vi "Save-OsciVsTime.vi"(0 "X-Values":dbl[](array[numeric]) format="%.2f", 2 "error in":errorcluster, 3 "Y-Values":dbl[](array[numeric]) format="%.2f", 4 "comment":string, 5 "refnum":refnum<file>) -> (1 "error out":errorcluster)   [LabVIEW 2017]
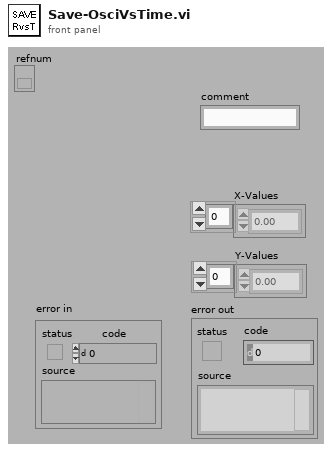
[diagram p1: front panel]
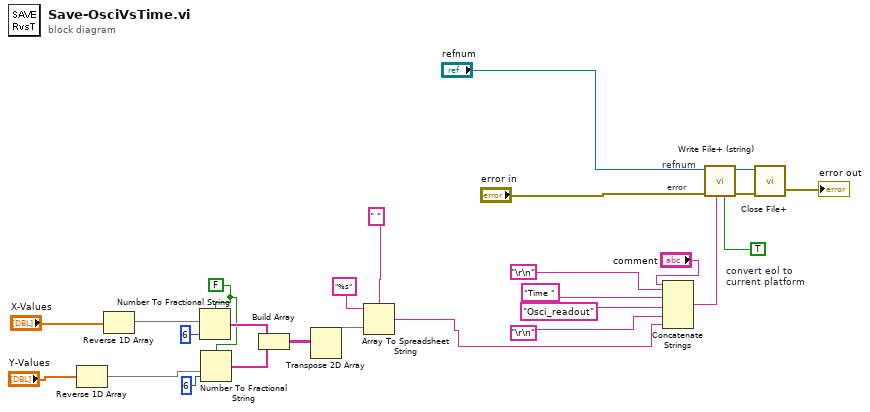
[diagram p0: block diagram]
diagram:
  w1 = FALSE
  w23 = TRUE  # convert eol to current platform
  # "error"
  # "refnum"
  n1 = Reverse 1D Array(array="Y-Values") -> (reversed array=w9:dbl[])
  n2 = Reverse 1D Array(array="X-Values") -> (reversed array=w8:dbl[])
  n3 = Number To Fractional String(use system decimal point (T)=w1, number=w8, precision (6)=i16 6) -> (F-format string=w19:string[])  [unwired: 1 out]
  n4 = Number To Fractional String(use system decimal point (T)=w1, number=w9, precision (6)=i16 6) -> (F-format string=w18:string[])  [unwired: 1 in]
  n5 = Build Array(w19, w18) -> (w17:string[][])
  n6 = Transpose 2D Array(2D array=w17) -> (transposed array=w16:string[][])
  n7 = Array To Spreadsheet String(delimiter (Tab)=" ", array=w16, 3:"%s" ("format (%.3f)")) -> (spreadsheet string=w2:string)
  n8 = Concatenate Strings("comment", "\r\n", "Time ", "Osci_readout", "\r\n", w2) -> (w20:string)
  n9 = call <vilib>:"Write File+ (string).vi"("convert eol? (no:F)"=w23, "string"=w20, "error in (no error)"="error in", "refnum"="refnum") -> ("error out"=w25:errorcluster, "dup refnum"=w24:refnum<file>)  [unwired: 2 in, 2 out]
  n10 = call <vilib>:"Close File+.vi"("error in (no error)"=w25, "refnum"=w24) -> ("error out"=→"error out":errorcluster)  [unwired: 5 out]
